vi "Unflatten Value.vi"(0 "Tree Data In":refnum<class "Tree Data.lvclass">, 7 "Value":string, 11 "Error In":errorcluster) -> (4 "Tree Data Out":refnum<class "Tree Data.lvclass">, 15 "Error Out":errorcluster)   [LabVIEW 2016, in "Tree Data.lvclass"]
uses:
  Tree Data.lvclass
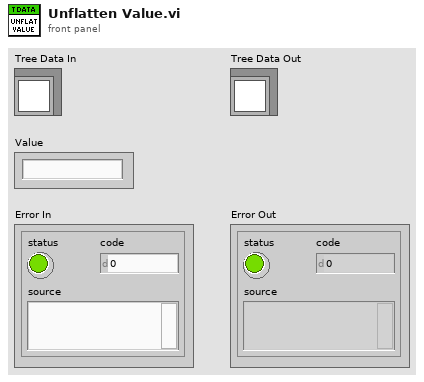
[diagram p1: front panel]
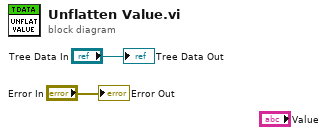
[diagram p0: block diagram]
diagram:
  "Tree Data Out" <- "Tree Data In"
  "Error Out" <- "Error In"
